vi "FileIO-Update Parameter File Presets Hierarchically.vi"(0 "Presets":refnum<vi>, 7 "folder":path, 11 "selected":path) -> ()   [LabVIEW 2020]
uses:
  Controls/KMultilevel Ring/KMultilevel Ring.xctl
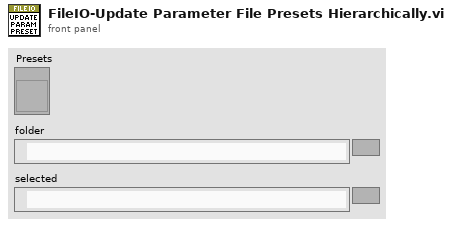
[diagram p1: front panel]
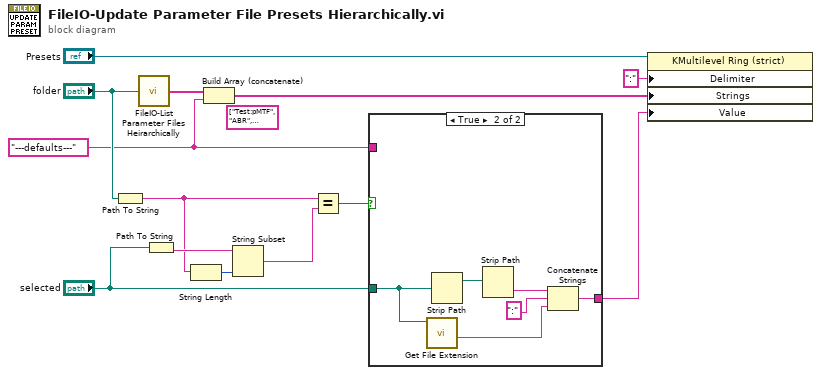
[diagram p0: block diagram]
diagram:
  (unwired) string[] ["Test:pMTF", "ABR", "pMTF", "--- defaults ---"] ("appended array")
  w1 = "---defaults---"
  n1 = Path To String(path="folder") -> (string=w7:string)
  n2 = call "FileIO-List Parameter Files Heirarchically.vi"("folder"="folder") -> ("Parameter file names"=w13:string[])  [unwired: 14 in]
  n3 = Path To String(path="selected") -> (string=w8:string)
  n4 = String Length(string=w7) -> (length=w5:i32)
  n5 = Build Array (concatenate)(w13, w1) -> (w10:string[])
  n6 = String Subset(string=w8, length (rest)=w5) -> (substring=w6:string)  [unwired: 1 in]
  n7 = Equal?(x=w7, y=w6) -> (x = y?=w2:bool)
  n8 = case shown="True" w2 {
    tunnel: "selected" -> [_ w20]
    tunnel: [w14 w15] -> w3
    tunnel: w1 -> [w14 _]
    frame False {
    }
    frame True {
      n9 = call <vilib>:"Get File Extension.vi"("file"=w20) -> ("filename without extension"=w16:string)  [unwired: 6 in, 4 out]
      n10 = Strip Path(path=w20) -> (stripped path=w19:path)  [unwired: 1 out]
      n11 = Strip Path(path=w19) -> (name=w18:string)  [unwired: 1 out]
      n12 = Concatenate Strings(w18, ":", w16) -> (w15:string)
    }
  }
  n13 = property class="KMultilevel Ring (strict)"(reference="Presets", "Delimiter"=":", "Strings"=w10, "Value"=w3) -> ()  [unwired: 1 in, 2 out]
